vi "Main.vi"() -> ()   [LabVIEW 2014]
uses:
  <vilib>/Utility/sysdir.llb/System Directory Type.ctl
  DataTypedef.ctl
panel:
  out "Cluster":T1
  in  "Load":bool
  in  "Save":bool
  in  "String 3":string
  in  "String 2":string
  in  "String 1":string
  in  "String 0":string
  in  "Slide 3":bool
  in  "Slide 2":bool
  in  "Slide 1":bool
  in  "Slide 0":bool
  in  "Numeric 3":dbl
  in  "Numeric 2":dbl
  in  "Numeric 1":dbl
  in  "Numeric 0":dbl
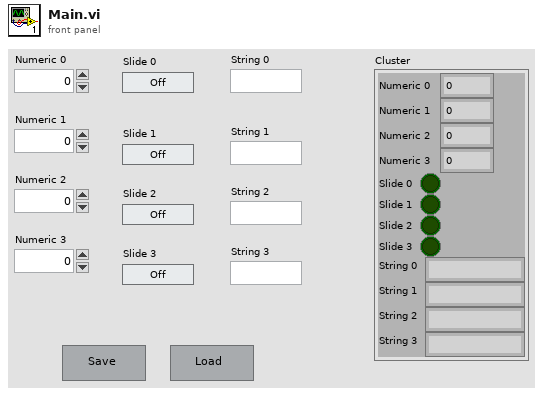
[diagram p1: front panel]
types:
  T1 = cluster{"Numeric 0":dbl, "Numeric 1":dbl, "Numeric 2":dbl, "Numeric 3":dbl, "Slide 0":bool, "Slide 1":bool, "Slide 2":bool, "Slide 3":bool, "String 0":string, "String 1":string, "String 2":string, "String 3":string}
  T2 = typedef "DataTypedef.ctl" = cluster{"Numeric 0":dbl, "Numeric 1":dbl, "Numeric 2":dbl, "Numeric 3":dbl, "Slide 0":bool, "Slide 1":bool, "Slide 2":bool, "Slide 3":bool, "String 0":string, "String 1":string, "String 2":string, "String 3":string}
  T3 = typedef "System Directory Type.ctl" = i32
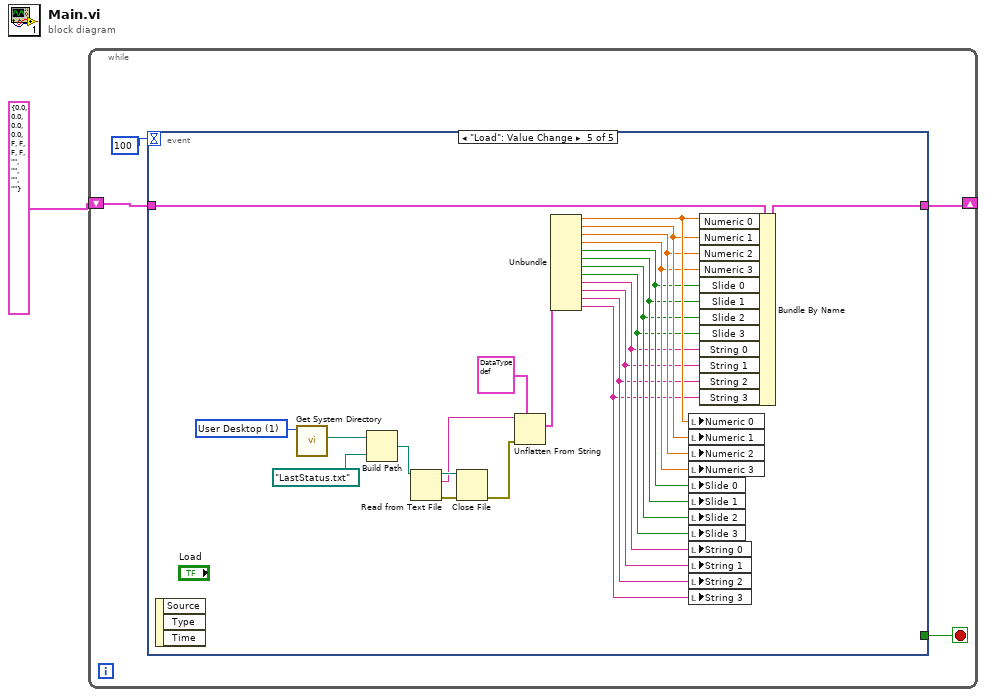
[diagram p0: block diagram]
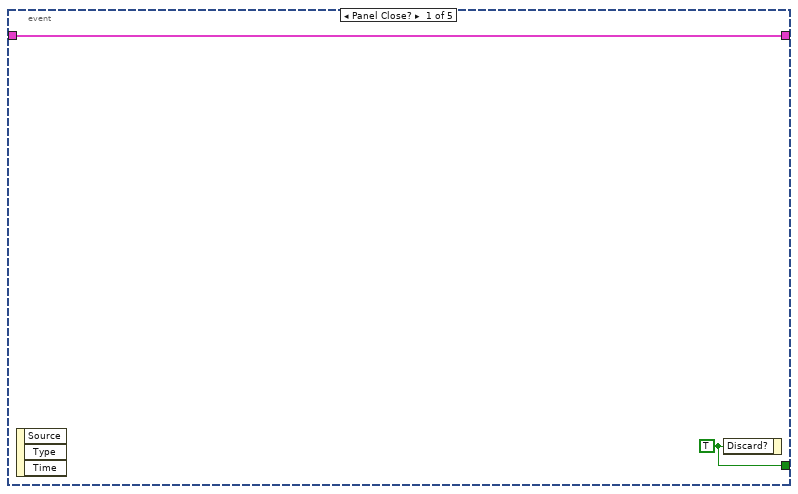
[diagram p2: hidden frame]
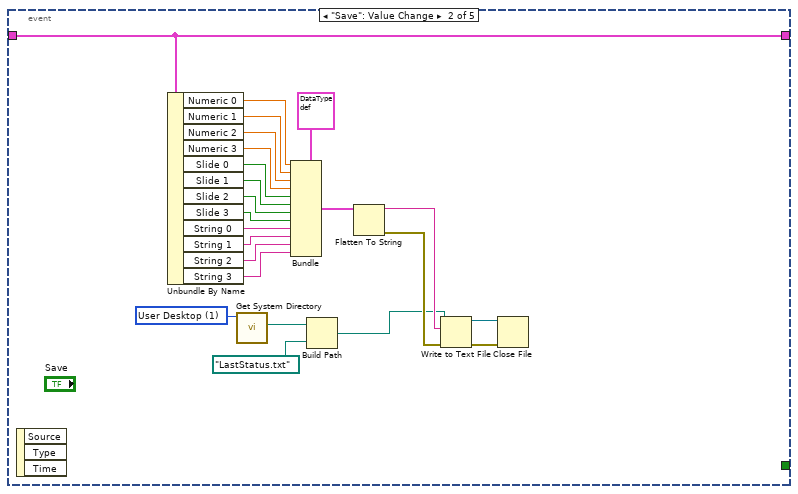
[diagram p3: hidden frame]
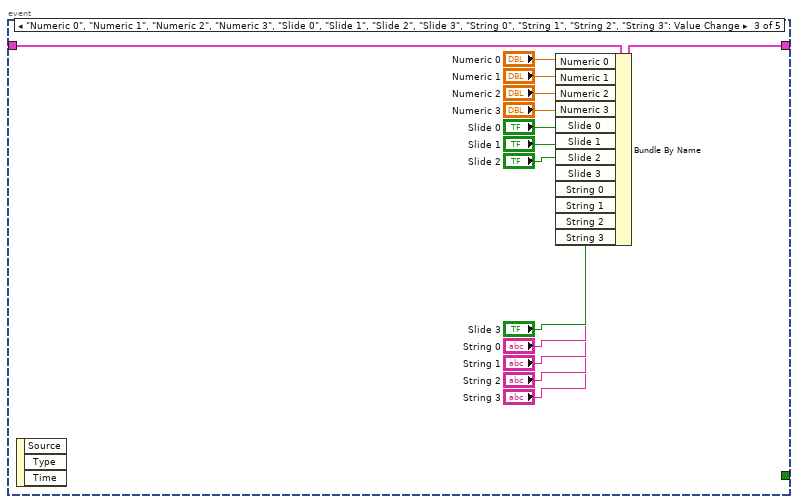
[diagram p4: hidden frame]
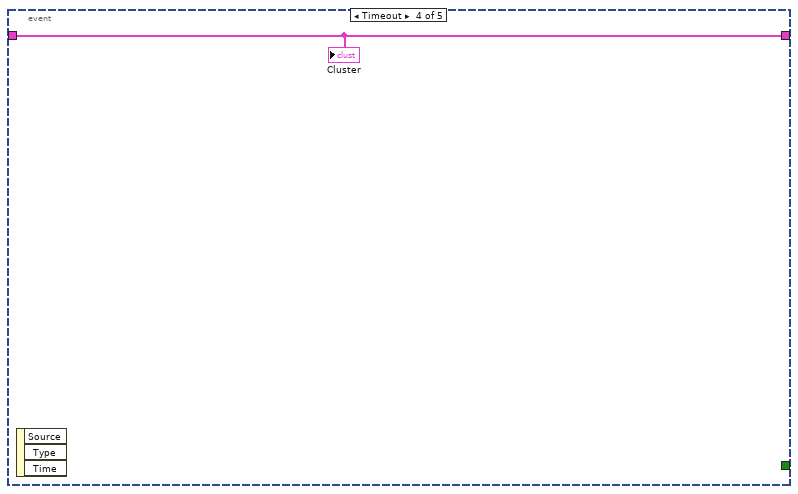
[diagram p5: hidden frame]
diagram:
  n1 = while {
    shift-right: [w4] -> _
    shift-left: T1 {"Numeric 0"=0.0, "Numeric 1"=0.0, "Numeric 2"=0.0, "Numeric 3"=0.0, "Slide 0"=FALSE, "Slide 1"=FALSE, "Slide 2"=FALSE, "Slide 3"=FALSE, "String 0"="", "String 1"="", "String 2"="", "String 3"=""} ("Cluster") -> [w3]
    stop <- w5 stop-if-true
    n2 = event shown="[4] \"Load\": Value Change" {
      selector: _ -> [_ _ _ _ _]
      dyn-events: _ -> [_ _ _ _ _]
      timeout: 100 -> [_ _ _ _ _]
      tunnel: [w7 _ _ _ _] -> w5
      tunnel: [w6 w30 w43 w45 w58] -> w4
      tunnel: w3 -> [w6 w30 w44 w45 w69]
      event Panel Close? {
        w7 = TRUE ("Discard?")
        n3 = event-data() -> ()  [unwired: 1 in, 3 out]
        n4 = event-data("Discard?"=w7) -> ()  [unwired: 1 in, 1 out]
      }
      event "Save": Value Change {
        w12 = T3 1 items=["User Home"=0, "User Desktop"=1, "User Documents"=2, "User Application Data"=3, "User Preferences"=4, "User Temporary"=5, "Public Documents"=6, "Public Application Data"=7, "Public Preferences"=8, "Public Cache"=13, "System Core Libraries"=9, "System Installed Libraries"=10, "Application Files"=11, "Boot Volume Root"=12] ("system directory type")
        n5 = event-data() -> ()  [unwired: 1 in, 3 out]
        n6 = Unbundle By Name(w30) -> ("Numeric 0"=w29:dbl, "Numeric 1"=w28:dbl, "Numeric 2"=w27:dbl, "Numeric 3"=w26:dbl, "Slide 0"=w25:bool, "Slide 1"=w24:bool, "Slide 2"=w23:bool, "Slide 3"=w22:bool, "String 0"=w21:string, "String 1"=w20:string, "String 2"=w19:string, "String 3"=w18:string)
        n7 = call <vilib>:"Get System Directory.vi"("system directory type"=w12) -> ("system directory"=w11:path)  [unwired: 10 in]
        n8 = Bundle(cluster=T2 {"Numeric 0"=0.0, "Numeric 1"=0.0, "Numeric 2"=0.0, "Numeric 3"=0.0, "Slide 0"=FALSE, "Slide 1"=FALSE, "Slide 2"=FALSE, "Slide 3"=FALSE, "String 0"="", "String 1"="", "String 2"="", "String 3"=""}, "Numeric 0"=w29, "Numeric 1"=w28, "Numeric 2"=w27, "Numeric 3"=w26, "Slide 0"=w25, "Slide 1"=w24, "Slide 2"=w23, "Slide 3"=w22, "String 0"=w21, "String 1"=w20, "String 2"=w19, "String 3"=w18) -> (w17:T2)
        n9 = Build Path(base path=w11, name or relative path=path "LastStatus.txt") -> (appended path=w9:path)
        n10 = Flatten To String(anything=w17) -> (data string=w16:string, error out=w15:errorcluster)  [unwired: 3 in, 1 out]
        n11 = Write to Text File(file (use dialog)=w9, text=w16, error in=w15) -> (refnum out=w13:refnum<file>, error out=w14:errorcluster)  [unwired: 1 in, 1 out]
        n12 = Close File(refnum=w13, error in=w14) -> ()  [unwired: 2 out]
      }
      event "Numeric 0", "Numeric 1", "Numeric 2", "Numeric 3", "Slide 0", "Slide 1", "Slide 2", "Slide 3", "String 0", "String 1", "String 2", "String 3": Value Change {
        n13 = event-data() -> ()  [unwired: 1 in, 3 out]
        n14 = Bundle By Name(cluster=w44, "Numeric 0"="Numeric 0", "Numeric 1"="Numeric 1", "Numeric 2"="Numeric 2", "Numeric 3"="Numeric 3", "Slide 0"="Slide 0", "Slide 1"="Slide 1", "Slide 2"="Slide 2", "Slide 3"="Slide 3", "String 0"="String 0", "String 1"="String 1", "String 2"="String 2", "String 3"="String 3") -> (w43:T1)
      }
      event Timeout {
        n15 = event-data() -> ()  [unwired: 1 in, 3 out]
        "Cluster" <- w45
      }
      event "Load": Value Change {
        w66 = T3 1 items=["User Home"=0, "User Desktop"=1, "User Documents"=2, "User Application Data"=3, "User Preferences"=4, "User Temporary"=5, "Public Documents"=6, "Public Application Data"=7, "Public Preferences"=8, "Public Cache"=13, "System Core Libraries"=9, "System Installed Libraries"=10, "Application Files"=11, "Boot Volume Root"=12] ("system directory type")
        n16 = event-data() -> ()  [unwired: 1 in, 3 out]
        n17 = call <vilib>:"Get System Directory.vi"("system directory type"=w66) -> ("system directory"=w65:path)  [unwired: 10 in]
        n18 = Build Path(base path=w65, name or relative path=path "LastStatus.txt") -> (appended path=w63:path)
        n19 = Read from Text File(file (use dialog)=w63) -> (refnum out=w67:refnum<file>, text=w61:string, error out=w68:errorcluster)  [unwired: 3 in, 1 out]
        n20 = Close File(refnum=w67, error in=w68) -> (error out=w62:errorcluster)  [unwired: 1 out]
        n21 = Unflatten From String(type=T2 {"Numeric 0"=0.0, "Numeric 1"=0.0, "Numeric 2"=0.0, "Numeric 3"=0.0, "Slide 0"=FALSE, "Slide 1"=FALSE, "Slide 2"=FALSE, "Slide 3"=FALSE, "String 0"="", "String 1"="", "String 2"="", "String 3"=""} ("cluster"), binary string=w61, error in (no error)=w62) -> (value=w59:T2)  [unwired: 2 in, 2 out]
        n22 = Unbundle(w59) -> ("Numeric 0"=w57:dbl, "Numeric 1"=w56:dbl, "Numeric 2"=w55:dbl, "Numeric 3"=w54:dbl, "Slide 0"=w53:bool, "Slide 1"=w52:bool, "Slide 2"=w51:bool, "Slide 3"=w50:bool, "String 0"=w49:string, "String 1"=w48:string, "String 2"=w47:string, "String 3"=w46:string)
        n23 = local write "Numeric 0"(w57) -> ()
        n24 = local write "Numeric 1"(w56) -> ()
        n25 = local write "Numeric 2"(w55) -> ()
        n26 = local write "Numeric 3"(w54) -> ()
        n27 = local write "Slide 0"(w53) -> ()
        n28 = local write "Slide 1"(w52) -> ()
        n29 = local write "Slide 2"(w51) -> ()
        n30 = local write "Slide 3"(w50) -> ()
        n31 = local write "String 0"(w49) -> ()
        n32 = local write "String 1"(w48) -> ()
        n33 = local write "String 2"(w47) -> ()
        n34 = local write "String 3"(w46) -> ()
        n35 = Bundle By Name(cluster=w69, "Numeric 0"=w57, "Numeric 1"=w56, "Numeric 2"=w55, "Numeric 3"=w54, "Slide 0"=w53, "Slide 1"=w52, "Slide 2"=w51, "Slide 3"=w50, "String 0"=w49, "String 1"=w48, "String 2"=w47, "String 3"=w46) -> (w58:T1)
      }
    }
  }
